vi "encoder_test_3mode_2motor_v1.vi"() -> ()   [LabVIEW 2014]
uses:
  <vilib>/rvi/FXPMathLib/FxpSinAndCos/subVIs/nifxpmath_SinAndCos_SimConfig.ctl
  <vilib>/rvi/Emulation/niFpgaGetClockAttributes.vi
  <vilib>/rvi/Emulation/niFpgaSctlEmulationGetInTimedLoop.vi
  <vilib>/rvi/Emulation/niFpgaEmulationReportErrorSimple.vi
  <vilib>/rvi/eio/common/nirviEmuTemplateMethod_errors.vi
  <vilib>/rvi/Emulation/niFpgaProcessEmulError.vi
  <vilib>/rvi/Emulation/niFpgaCriticalErrorInLSC.vi
  <vilib>/rvi/FXPMathLib/FxpSinAndCos/simVIs/DllFxpSinAndCosTemp_sub.vi
  <vilib>/rvi/interface/RandomDataEmulation/nirviRandomDataMultiElementFPGAFIFO.vi
  <instcachedir>/0/nirviRandomDataMultiElementFPGAFIFO_AD0CFC12EF974623A9C2E4184BC062B2.lvgen/nirviRandomDataMultiElementFPGAFIFO_AD0CFC12EF974623A9C2E4184BC062B2_020.vi
  <vilib>/rvi/interface/RandomDataEmulation/niFpgaRandomDataHandleErrors.vi
  <vilib>/eio/EIONode/EIONode.xnode
  <vilib>/rvi/FXPMathLib/FxpMul/XNode/nifxpmath_Multiplier.xnode
  <vilib>/rvi/FXPMathLib/FxpSinAndCos/XNode/nifxpmath_SinAndCos.xnode
  <vilib>/rvi/Analysis/measure/butterworth/XNode/niFpgaButterworthFilter.xnode
  <vilib>/rvi/FXPMathLib/FxpSub/XNode/nifxpmath_Sub.xnode
  <vilib>/rvi/FXPMathLib/FxpAdd/XNode/nifxpmath_Add.xnode
  <vilib>/rvi/DataTransferAndStorage/Container/XNode/niFpgaContainer.xnode
  <vilib>/rvi/interface/RandomDataEmulation/nirviRandomDataFpgaMultiElementTemplate.vi
  <vilib>/rvi/FXPMathLib/sim/FxpSim.dll
panel:
  out "Dy_d (mm/s)":fxp<+,64,32>
  out "omega_y (rad/s)":fxp<+/-,64,35>
  in  "Velocity Estimation_y":i16(ring) items=["Step", "Ramp", "Sine"]
  out "Dy_d (T)":fxp<+/-,46,10>
  out "mt 2":u32
  out "omega_y (T)":fxp<+/-,20,9>
  out "omega_y (M)":fxp<+/-,64,30>
  out "Dy_d (M)":fxp<+/-,64,27>
  in  "Dy_d_M_Tc (mSec)":u32 format="%#_6f"
  out "omega_y(M_avg)":fxp<+/-,64,35>
  out "Dy_d (M_avg)":fxp<+,64,32>
  in  "Dy_d_M_avg_Tc (uSec)":u32 caption="Count(uSec)"
  out "rad_y(NrTheta)":fxp<+/-,48,33>
  out "Dy (mm)":fxp<+/-,56,32>
  out "Encoder Position_y":i32
  in  "Encoder Reset_y":bool
  out "omega_p (M_avg)":fxp<+/-,64,35>
  out "Dp_d (M_avg)":fxp<+/-,64,32>
  in  "Dp_d_M_avg_Tc (uSec)":u32 caption="D_d_M_avg_Tc (uSec)"
  out "omega_p (M)":fxp<+/-,64,30>
  out "Dp_d (M)":fxp<+/-,64,27>
  in  "Dp_d_M_Tc (mSec)":u32 format="%#_6f"
  out "Dp_d (T)":fxp<+/-,46,10>
  out "omega_p(T)":fxp<+/-,20,9>
  in  "Velocity Estimation_p":i16(ring) items=["M_avg method", "M method", "T method"]
  out "Dpr_ramp":fxp<+/-,64,30>
  out "Dpr_slope":fxp<+/-,33,17>
  in  "Dpr_time":fxp<+/-,16,11>
  out "Dpr_sin":fxp<+/-,28,11>
  out "Dpr_sin_d":fxp<+/-,64,16>
  out "Dpr_sin_dd":fxp<+/-,64,25>
  out "Sin omega_p":fxp<+/-,41,8>
  in  "Sin offset_p":fxp<+/-,27,10>
  in  "Sin magnitude_p":fxp<+/-,11,8>
  in  "Sin wave frequency_p (Hz)":fxp<+/-,21,5>
  out "Time now (s)":fxp<+,52,14>
  out "Dpr":fxp<+/-,64,31>
  in  "Dpr_end":fxp<+/-,16,11>
  in  "Command type_p":i16(ring) items=["Step", "Ramp", "Sine"]
  out "Dp_i":fxp<+/-,34,18>
  in  "Dp_tolorence":fxp<+/-,14,3>
  in  "Ki_p":fxp<+/-,20,6>
  out "Dp_error":fxp<+/-,24,11>
  in  "Direction":bool
  out "Fmr_p":fxp<+/-,64,31>
  in  "Kd_p":fxp<+/-,20,8>
  in  "Kp_p":fxp<+/-,20,12>
  in  "scaled coefficients_Dp_dd":i32[](array[numeric])=[780119100, 146811362]
  out "Dp_dd":fxp<+/-,36,29>
  in  "Ini coe.":bool
  out "va_p":fxp<+/-,38,8>
  out "vb_p":fxp<+/-,38,8>
  in  "stop motor_p":bool
  out "vq_p":fxp<+/-,20,5> format="%.57g"
  out "vd_p":fxp<+/-,20,5>
  out "Dp_d (mm/s)":fxp<+/-,32,12>
  out "mt":u32
  out "omega_p (rad/s)":fxp<+/-,32,18>
  in  "mt0":u32
  out "Dp (mm)":fxp<+/-,22,7>
  out "rad_p(NrTheta)":fxp<+/-,33,18>
  out "Encoder Position_p":i32
  in  "Encoder Reset_p":bool
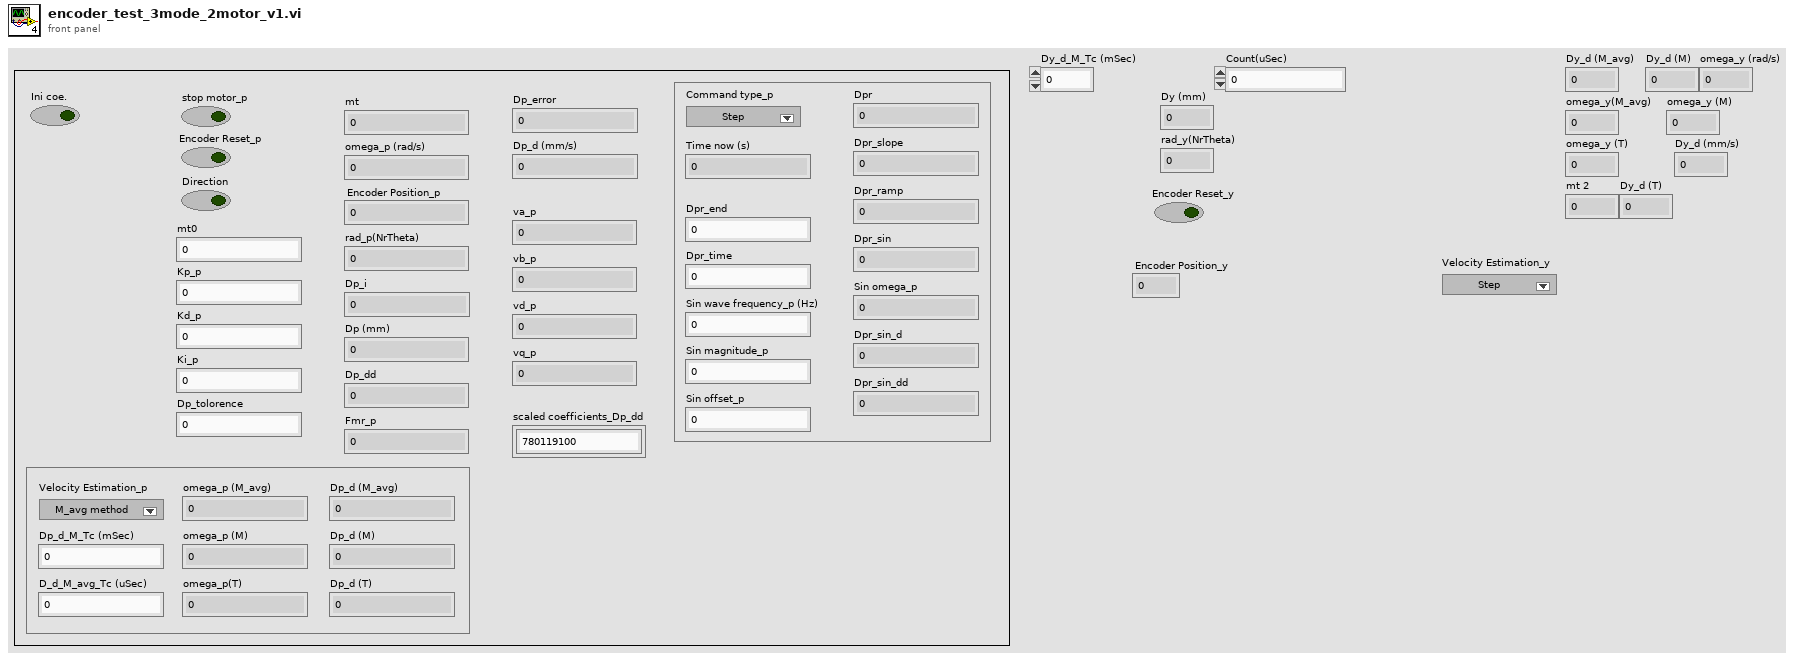
[diagram p1: front panel]
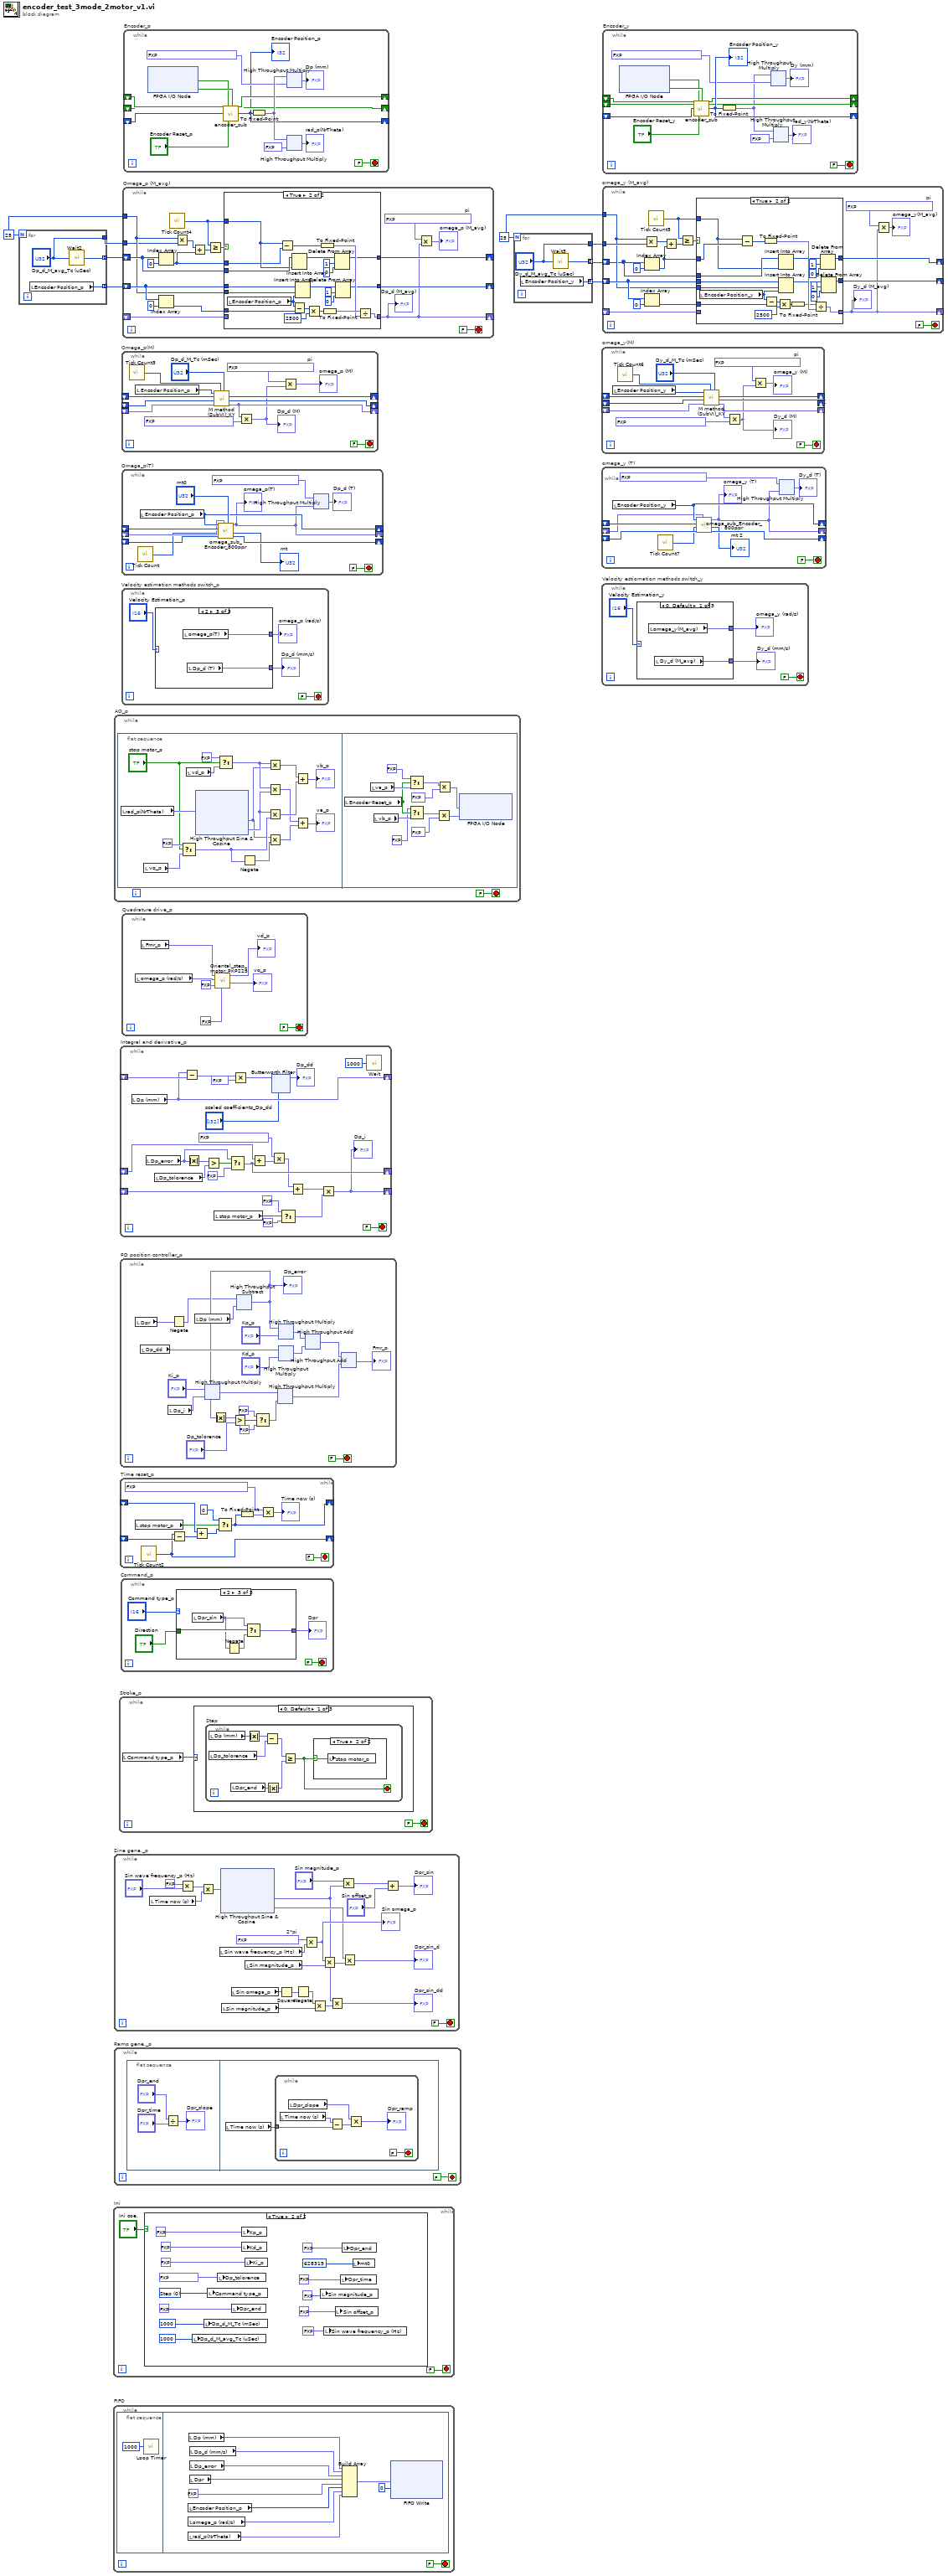
[diagram p0: block diagram]
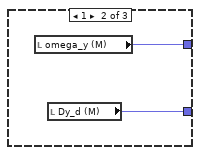
[diagram p2: hidden frame]
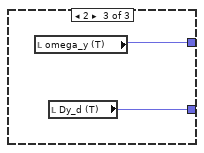
[diagram p3: hidden frame]
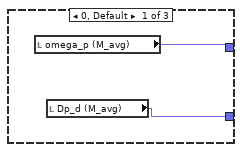
[diagram p6: hidden frame]
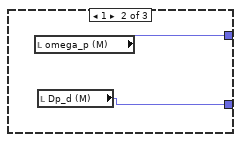
[diagram p7: hidden frame]
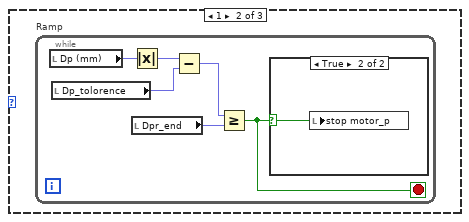
[diagram p9: hidden frame]
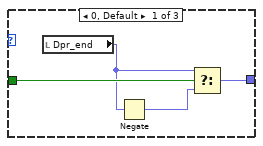
[diagram p12: hidden frame]
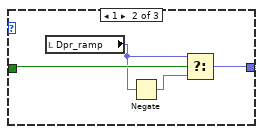
[diagram p13: hidden frame]
diagram:
  w4 = 25
  w8 = 25
  n1 = for {
    N: w8 -> [_]
    tunnel: ["Dp_d_M_avg_Tc (uSec)"] -> w5
    tunnel: [w10] -> w7 mode=indexing
    tunnel: [w9] -> w6 mode=indexing
    n2 = local read "Encoder Position_p"() -> (w9:i32)
    n3 = call "Wait2"("Count(uSec)"="Dp_d_M_avg_Tc (uSec)") -> ("Tick Count(uSec)"=w10:u32)
  }
  n4 = while "Ini" {
    stop <- FALSE stop-if-true
    n5 = case shown="True" "Ini coe." {
      frame False {
      }
      frame True {
        w21 = i16 0 items=["Step", "Ramp", "Sine"] ("Command type")
        n6 = local write "Dp_d_M_avg_Tc (uSec)"(u32 1000 ("D_d_M_avg_Tc (uSec)")) -> ()
        n7 = local write "Dp_d_M_Tc (mSec)"(u32 1000 ("D_d_M_Tc (uSec)")) -> ()
        n8 = local write "Command type_p"(w21) -> ()
        n9 = local write "Dp_tolorence"(fxp<+/-,14,3> 0.009765625 ("D_tolorence")) -> ()
        n10 = local write "Dpr_end"(fxp<+/-,16,11> 20.0 ("Dr_end")) -> ()
        n11 = local write "Kp_p"(fxp<+/-,20,12> 10.0 ("Kp")) -> ()
        n12 = local write "Kd_p"(fxp<+/-,20,8> 2.0 ("Kd")) -> ()
        n13 = local write "Ki_p"(fxp<+/-,20,6> 8.0 ("D_i")) -> ()
        n14 = local write "Sin magnitude_p"(fxp<+/-,11,8> 20.0 ("Sin magnitude")) -> ()
        n15 = local write "Sin wave frequency_p (Hz)"(fxp<+/-,21,5> 0.5 ("Sin wave frequency (Hz)")) -> ()
        n16 = local write "Sin offset_p"(fxp<+/-,27,10> 0.0 ("Sin offset")) -> ()
        n17 = local write "Dpr_time"(fxp<+/-,16,11> 5.0 ("Dr_time")) -> ()
        n18 = local write "Dpr_end"(fxp<+/-,11,7> 20.0 ("Fmr")) -> ()
        n19 = local write "mt0"(u32 628319 ("mt0")) -> ()
      }
    }
  }
  n20 = while "FIFO" {
    stop <- FALSE stop-if-true
    n21 = flat-sequence {
      frame #0 {
        n22 = call "Loop Timer"("Count(uSec)"=u32 1000) -> ()  [unwired: 1 out]
      }
      frame #1 {
        n23 = local read "Encoder Position_p"() -> (w33:i32)
        n24 = local read "omega_p (rad/s)"() -> (w32:fxp<+/-,32,18>)
        n25 = local read "rad_p(NrTheta)"() -> (w31:fxp<+/-,33,18>)
        n26 = local read "Dp (mm)"() -> (w37:fxp<+/-,22,7>)
        n27 = local read "Dp_d (mm/s)"() -> (w36:fxp<+/-,32,12>)
        n28 = local read "Dp_error"() -> (w35:fxp<+/-,24,11>)
        n29 = local read "Dpr"() -> (w34:fxp<+/-,64,31>)
        n30 = Build Array(w37, w36, w35, w34, fxp<+/-,64,32> 0.0 ("element"), w33, w32, w31) -> (w38:fxp<+/-,64,32>[])
        n31 = xnode ("FIFO Write")("Element"=w38, "Timeout"=0) -> ()  [unwired: 1 in, 2 out]
      }
    }
  }
  n32 = while "Sine gene._p" {
    stop <- FALSE stop-if-true
    w57 = fxp<+,20,3> 6.2831878662109375  # 2*pi
    n33 = local read "Time now (s)"() -> (w60:fxp<+,52,14>)
    n34 = Multiply(x=fxp<+,1,2> 2.0, y="Sin wave frequency_p (Hz)") -> (x*y=w61:fxp<+/-,21,6>)
    n35 = Multiply(x=w61, y=w60) -> (x*y=w41:fxp<+/-,64,20>)
    n36 = local read "Sin wave frequency_p (Hz)"() -> (w56:fxp<+/-,21,5>)
    n37 = xnode "High Throughput Sine & Cosine"("x (pi)"=w41) -> ("sin(x)"=w45:fxp<+/-,16,2>, "cos(x)"=w52:fxp<+/-,16,2>)
    n38 = local read "Sin magnitude_p"() -> (w47:fxp<+/-,11,8>)
    n39 = local read "Sin omega_p"() -> (w48:fxp<+/-,41,8>)
    n40 = local read "Sin magnitude_p"() -> (w51:fxp<+/-,11,8>)
    n41 = Square(x=w48) -> (x^2=w49:fxp<+,64,14>)
    n42 = Negate(x=w49) -> (-x=w46:fxp<+/-,64,15>)
    n43 = Multiply(x=w57, y=w56) -> (x*y=w53:fxp<+/-,41,8>)
    "Sin omega_p" <- w53
    n44 = Multiply(x=w46, y=w47) -> (x*y=w50:fxp<+/-,64,23>)
    n45 = Multiply(x=w53, y=w51) -> (x*y=w58:fxp<+/-,51,15>)
    n46 = Multiply(x=w45, y=w50) -> (x*y=→"Dpr_sin_dd":fxp<+/-,64,25>)
    n47 = Multiply(x="Sin magnitude_p", y=w45) -> (x*y=w59:fxp<+/-,27,10>)
    n48 = Multiply(x=w52, y=w58) -> (x*y=→"Dpr_sin_d":fxp<+/-,64,16>)
    n49 = Add(x=w59, y="Sin offset_p") -> (x+y=→"Dpr_sin":fxp<+/-,28,11>)
  }
  n50 = while "Ramp gene._p" {
    stop <- FALSE stop-if-true
    n51 = flat-sequence {
      frame #0 {
        n52 = Divide(x="Dpr_end", y="Dpr_time") -> (x/y=→"Dpr_slope":fxp<+/-,33,17>)
      }
      frame #1 {
        n53 = local read "Time now (s)"() -> (w98:fxp<+,52,14>)
        n54 = while {
          tunnel: w98 -> [w104]
          stop <- FALSE stop-if-true
          n55 = local read "Time now (s)"() -> (w101:fxp<+,52,14>)
          n56 = local read "Dpr_slope"() -> (w102:fxp<+/-,33,17>)
          n57 = Subtract(x=w101, y=w104) -> (x-y=w103:fxp<+/-,53,15>)
          n58 = Multiply(x=w102, y=w103) -> (x*y=→"Dpr_ramp":fxp<+/-,64,30>)
        }
      }
    }
  }
  n59 = while "AO_p" {
    stop <- FALSE stop-if-true
    n60 = flat-sequence {
      frame #0 {
        n61 = local read "rad_p(NrTheta)"() -> (w121:fxp<+/-,33,18>)
        n62 = local read "vq_p"() -> (w119:fxp<+/-,20,5>)
        n63 = Select(t=fxp<+,20,5> 0.0, s="stop motor_p", f=w119) -> (s? t:f=w116:fxp<+/-,21,6>)
        n64 = local read "vd_p"() -> (w120:fxp<+/-,20,5>)
        n65 = xnode "High Throughput Sine & Cosine"("x (pi)"=w121) -> ("sin(x)"=w112:fxp<+/-,17,2>, "cos(x)"=w114:fxp<+/-,17,2>)
        n66 = Select(t=fxp<+,20,5> 0.0, s="stop motor_p", f=w120) -> (s? t:f=w113:fxp<+/-,21,6>)
        n67 = Negate(x=w116) -> (-x=w115:fxp<+/-,21,6>)
        n68 = Multiply(x=w113, y=w112) -> (x*y=w111:fxp<+/-,37,7>)
        n69 = Multiply(x=w113, y=w114) -> (x*y=w109:fxp<+/-,37,7>)
        n70 = Multiply(x=w114, y=w116) -> (x*y=w110:fxp<+/-,37,7>)
        n71 = Multiply(x=w112, y=w115) -> (x*y=w108:fxp<+/-,37,7>)
        n72 = Add(x=w111, y=w110) -> (x+y=→"vb_p":fxp<+/-,38,8>)
        n73 = Add(x=w109, y=w108) -> (x+y=→"va_p":fxp<+/-,38,8>)
      }
      frame #1 {
        n74 = local read "Encoder Reset_p"() -> (w155:bool)
        n75 = local read "va_p"() -> (w157:fxp<+/-,38,8>)
        n76 = local read "vb_p"() -> (w156:fxp<+/-,38,8>)
        n77 = Select(t=fxp<+/-,20,5> 5.0 ("y"), s=w155, f=w157) -> (s? t:f=w158:fxp<+/-,38,8>)
        n78 = Select(t=fxp<+/-,20,5> 0.0 ("y"), s=w155, f=w156) -> (s? t:f=w159:fxp<+/-,38,8>)
        n79 = Multiply(x=w159, y=fxp<+/-,20,5> -0.5) -> (x*y=w163:fxp<+/-,57,12>)
        n80 = Multiply(x=w158, y=fxp<+/-,20,5> -0.5) -> (x*y=w162:fxp<+/-,57,12>)
        n81 = xnode "FPGA I/O Node"("Mod8/AO0"=w162, "Mod8/AO1"=w163) -> ()  [unwired: 2 in, 2 out]
      }
    }
  }
  n82 = while "Stroke_p" {
    stop <- FALSE stop-if-true
    n83 = local read "Command type_p"() -> (w165:i16)
    n84 = case shown="0, Default" w165 {
      frame 0, Default {
        n85 = while "Step" {
          stop <- w166 stop-if-true
          n86 = local read "Dp_tolorence"() -> (w168:fxp<+/-,14,3>)
          n87 = local read "Dp (mm)"() -> (w170:fxp<+/-,22,7>)
          n88 = local read "Dpr_end"() -> (w172:fxp<+/-,16,11>)
          n89 = Absolute Value(x=w170) -> (abs(x)=w169:fxp<+,22,7>)
          n90 = Subtract(x=w169, y=w168) -> (x-y=w167:fxp<+/-,23,8>)
          n91 = Absolute Value(x=w172) -> (abs(x)=w171:fxp<+,16,11>)
          n92 = Greater Or Equal?(x=w167, y=w171) -> (x >= y?=w166:bool)
          n93 = case shown="True" w166 {
            selector: w166 -> [_ w173]
            frame False {
            }
            frame True {
              n94 = local write "stop motor_p"(w173) -> ()
            }
          }
        }
      }
      frame 1 {
        n95 = while "Ramp" {
          stop <- w174 stop-if-true
          n96 = local read "Dp (mm)"() -> (w176:fxp<+/-,22,7>)
          n97 = local read "Dp_tolorence"() -> (w178:fxp<+/-,14,3>)
          n98 = Absolute Value(x=w176) -> (abs(x)=w177:fxp<+,22,7>)
          n99 = local read "Dpr_end"() -> (w175:fxp<+/-,16,11>)
          n100 = Subtract(x=w177, y=w178) -> (x-y=w179:fxp<+/-,23,8>)
          n101 = Greater Or Equal?(x=w179, y=w175) -> (x >= y?=w174:bool)
          n102 = case shown="True" w174 {
            selector: w174 -> [_ w180]
            frame False {
            }
            frame True {
              n103 = local write "stop motor_p"(w180) -> ()
            }
          }
        }
      }
      frame 2 {
      }
    }
  }
  n104 = while "Integral and derivative_p" {
    shift-right: [w201] -> _
    shift-left: _ -> [w205]
    shift-right: [w191] -> _
    shift-left: _ -> [w192]
    shift-right: [w181] -> _
    shift-left: _ -> [w185]
    stop <- FALSE stop-if-true
    n105 = local read "Dp (mm)"() -> (w201:fxp<+/-,22,7>)
    n106 = local read "Dp_error"() -> (w193:fxp<+/-,24,11>)
    n107 = local read "Dp_tolorence"() -> (w196:fxp<+/-,14,3>)
    n108 = Subtract(x=w201, y=w205) -> (x-y=w204:fxp<+/-,23,8>)
    n109 = Absolute Value(x=w193) -> (abs(x)=w197:fxp<+,24,11>)
    n110 = Greater?(x=w197, y=w196) -> (0:w195:bool)
    n111 = local read "stop motor_p"() -> (w188:bool)
    n112 = Select(t=w193, s=w195, f=fxp<+,24,11> 0.0) -> (s? t:f=w191:fxp<+/-,25,12>)
    n113 = Multiply(x=w204, y=fxp<+/-,33,13> 1000.0) -> (x*y=w202:fxp<+/-,55,20>)
    n114 = Add(x=w192, y=w191) -> (x+y=w190:fxp<+/-,26,13>)
    n115 = Multiply(x=fxp<+/-,30,12> 0.000499725341796875, y=w190) -> (x*y=w184:fxp<+/-,55,24>)
    n116 = xnode "Butterworth Filter"("input data"=w202, "scaled coefficients"="scaled coefficients_Dp_dd") -> ("output data"=→"Dp_dd":fxp<+/-,36,24>)  [unwired: 1 in]
    n117 = Select(t=fxp<+,1,1> 0.0, s=w188, f=fxp<+,1,1> 1.0) -> (s? t:f=w182:fxp<+,1,1>)
    n118 = Add(x=w184, y=w185) -> (x+y=w183:fxp<+/-,32,16>)
    n119 = Multiply(x=w183, y=w182) -> (x*y=w181:fxp<+/-,32,16>)
    "Dp_i" <- w181
    n120 = call "Wait"("Count(uSec)"=u32 1000) -> ()  [unwired: 1 out]
  }
  n121 = while "PD position controller_p" {
    stop <- FALSE stop-if-true
    n122 = local read "Dpr"() -> (w216:fxp<+/-,64,31>)
    n123 = local read "Dp_dd"() -> (w232:fxp<+/-,36,29>)
    n124 = local read "Dp_i"() -> (w227:fxp<+/-,34,18>)
    n125 = Negate(x=w216) -> (-x=w215:fxp<+/-,64,32>)
    n126 = local read "Dp (mm)"() -> (w236:fxp<+/-,22,7>)
    n127 = xnode ("High Throughput Multiply")("x"="Ki_p", "y"=w227) -> ("x*y"=w221:fxp<+/-,54,24>)
    n128 = xnode "High Throughput Subtract"("x"=w215, "y"=w236) -> ("x-y"=w225:fxp<+/-,64,33>)
    "Dp_error" <- w225
    n129 = Absolute Value(x=w225) -> (abs(x)=w226:fxp<+,64,33>)
    n130 = Greater?(x=w226, y="Dp_tolorence") -> (0:w224:bool)
    n131 = Select(t=fxp<+,10,2> 1.0, s=w224, f=fxp<+,10,2> 0.0) -> (s? t:f=w220:fxp<+,10,2>)
    n132 = xnode ("High Throughput Multiply")("x"=w221, "y"=w220) -> ("x*y"=w217:fxp<+/-,64,26>)
    n133 = xnode ("High Throughput Multiply")("x"=w225, "y"="Kp_p") -> ("x*y"=w234:fxp<+/-,64,45>)
    n134 = xnode ("High Throughput Multiply")("x"=w232, "y"="Kd_p") -> ("x*y"=w233:fxp<+/-,56,37>)
    n135 = xnode ("High Throughput Add")("x"=w234, "y"=w233) -> ("x+y"=w218:fxp<+/-,64,46>)
    n136 = xnode ("High Throughput Add")("x"=w218, "y"=w217) -> ("x+y"=→"Fmr_p":fxp<+/-,64,47>)
  }
  n137 = while "Time reset_p" {
    shift-right: [w240] -> _
    shift-left: _ -> [w247]
    shift-right: [w242] -> _
    shift-left: _ -> [w243]
    stop <- FALSE stop-if-true
    n138 = local read "stop motor_p"() -> (w245:bool)
    n139 = call "Tick Count2"() -> ("Tick Count(uSec)"=w242:u32)
    n140 = Subtract(x=w242, y=w243) -> (x-y=w248:u32)
    n141 = Add(x=w247, y=w248) -> (x+y=w246:u32)
    n142 = Select(t=u32 0, s=w245, f=w246) -> (s? t:f=w240:u32)
    n143 = To Fixed-Point(number=w240) -> (fixed-point=w239:fxp<+,32,32>)  [unwired: 1 in]
    n144 = Multiply(x=fxp<+,20,-18> 1.0000003385357559e-06, y=w239) -> (x*y=→"Time now (s)":fxp<+,52,14>)
  }
  n145 = while "Command_p" {
    stop <- FALSE stop-if-true
    n146 = case shown="2" "Command type_p" {
      tunnel: [w253 w257 w261] -> w251
      tunnel: "Direction" -> [w256 w260 w264]
      frame 0, Default {
        n147 = local read "Dpr_end"() -> (w255:fxp<+/-,16,11>)
        n148 = Negate(x=w255) -> (-x=w254:fxp<+/-,17,12>)
        n149 = Select(t=w255, s=w256, f=w254) -> (s? t:f=w253:fxp<+/-,17,12>)
      }
      frame 1 {
        n150 = local read "Dpr_ramp"() -> (w258:fxp<+/-,64,30>)
        n151 = Negate(x=w258) -> (-x=w259:fxp<+/-,64,31>)
        n152 = Select(t=w258, s=w260, f=w259) -> (s? t:f=w257:fxp<+/-,64,31>)
      }
      frame 2 {
        n153 = local read "Dpr_sin"() -> (w262:fxp<+/-,28,11>)
        n154 = Negate(x=w262) -> (-x=w263:fxp<+/-,27,10>)
        n155 = Select(t=w262, s=w264, f=w263) -> (s? t:f=w261:fxp<+/-,28,11>)
      }
    }
    "Dpr" <- w251
  }
  n156 = while "Omega_p(M)" {
    shift-right: [w276] -> _
    shift-left: _ -> [w277]
    shift-right: [w272] -> _
    shift-left: _ -> [w273]
    shift-right: [w270] -> _
    shift-left: _ -> [w271]
    stop <- FALSE stop-if-true
    w267 = fxp<+/-,27,3> 3.1415926218032837  # pi
    n157 = call "Tick Count3"() -> ("Tick Count(mSec)"=w275:u32)
    n158 = local read "Encoder Position_p"() -> (w278:i32)
    n159 = call "M method (SubVI)_KY.vi"("Tc (mSec)"="Dp_d_M_Tc (mSec)", "Tick Count (mSec)"=w275, "Encoder velocity_pre (pulse/s)"=w271, "Shift Register in 2"=w273, "Shift Register in 1"=w277, "Encoder pulses"=w278) -> ("Encoder velocity (pulse/s)"=w270:fxp<+/-,64,32>, "Shift Register out 2"=w272:i32, "Shift Register out 1"=w276:u32)  [unwired: 3 in]
    n160 = Multiply(x=w270, y=fxp<+/-,20,-5> 0.002499997615814209) -> (x*y=w268:fxp<+/-,64,27>)
    "Dp_d (M)" <- w268
    n161 = Multiply(x=w267, y=w268) -> (x*y=→"omega_p (M)":fxp<+/-,64,30>)
  }
  n162 = while "Omega_p(T)" {
    shift-right: [w288] -> _
    shift-left: _ -> [w289]
    shift-right: [w281] -> _
    shift-left: _ -> [w287]
    shift-right: [w284] -> _
    shift-left: _ -> [w285]
    stop <- FALSE stop-if-true
    n163 = call "Tick Count"() -> ("Tick Count(Ticks)"=w286:u32)
    n164 = local read "Encoder Position_p"() -> (w288:i32)
    n165 = call "omega_sub_Encoder_800ppr.vi"("mt0"="mt0", "omega_pre"=w287, "ticks_m_pre"=w285, "ticks"=w286, "count_pre"=w289, "count"=w288) -> ("ticks_m"=w284:u32, "mt"=→"mt":u32, "omega"=w281:fxp<+/-,20,9>)  [unwired: 3 in]
    "omega_p(T)" <- w281
    n166 = xnode ("High Throughput Multiply")("x"=fxp<+/-,26,1> 0.3183099031448364, "y"=w281) -> ("x*y"=→"Dp_d (T)":fxp<+/-,46,10>)
  }
  n167 = while "Velocity estimation methods switch_p" {
    stop <- FALSE stop-if-true
    n168 = case shown="2" "Velocity Estimation_p" {
      tunnel: [w296 w298 w300] -> w293
      tunnel: [w295 w297 w299] -> w292
      frame 0, Default {
        n169 = local read "omega_p (M_avg)"() -> (w296:fxp<+/-,64,35>)
        n170 = local read "Dp_d (M_avg)"() -> (w295:fxp<+/-,64,32>)
      }
      frame 1 {
        n171 = local read "omega_p (M)"() -> (w298:fxp<+/-,64,30>)
        n172 = local read "Dp_d (M)"() -> (w297:fxp<+/-,64,27>)
      }
      frame 2 {
        n173 = local read "omega_p(T)"() -> (w300:fxp<+/-,20,9>)
        n174 = local read "Dp_d (T)"() -> (w299:fxp<+/-,46,10>)
      }
    }
    "Dp_d (mm/s)" <- w292
    "omega_p (rad/s)" <- w293
  }
  n175 = while "Quadrature drive_p" {
    stop <- FALSE stop-if-true
    n176 = local read "omega_p (rad/s)"() -> (w303:fxp<+/-,32,18>)
    n177 = local read "Fmr_p"() -> (w301:fxp<+/-,64,31>)
    n178 = call "Oriental_step_motor_PKP225.vi"("F_Threshold"=fxp<+,12,12> 10.0, "dFmr"=fxp<+/-,25,15> 0.0, "omega"=w303, "Fmr"=w301) -> ("vq_F"=→"vq_p":fxp<+/-,20,5>, "vd_F"=→"vd_p":fxp<+/-,20,5>)  [unwired: 6 in]
  }
  n179 = while "Omega_p (M_avg)" {
    tunnel: w8 -> [w319]
    shift-right: [w312] -> _
    shift-left: w7 -> [w323]
    shift-right: [w311] -> _
    shift-left: _ -> [w314]
    shift-right: [w313] -> _
    shift-left: w6 -> [w322]
    tunnel: w5 -> [w316]
    stop <- FALSE stop-if-true
    w310 = fxp<+/-,27,3> 3.1415926218032837  # pi
    n180 = Index Array(array=w323, index=0) -> (element=w317:u32)
    n181 = Index Array(array=w322, index=0) -> (element=w318:i32)
    n182 = call "Tick Count4"() -> ("Tick Count(uSec)"=w320:u32)
    n183 = Multiply(x=w319, y=w316) -> (x*y=w324:u32)
    n184 = Add(x=w324, y=w317) -> (x+y=w321:u32)
    n185 = Greater Or Equal?(x=w320, y=w321) -> (x >= y?=w315:bool)
    n186 = case shown="True" w315 {
      tunnel: w323 -> [w329 w346]
      tunnel: w322 -> [w328 w345]
      tunnel: w320 -> [_ w338]
      tunnel: w319 -> [_ w344]
      tunnel: w318 -> [_ w342]
      tunnel: w317 -> [_ w337]
      tunnel: w314 -> [w327 _]
      tunnel: [w328 w332] -> w313
      tunnel: [w329 w331] -> w312
      tunnel: [w327 w330] -> w311
      frame False {
      }
      frame True {
        n187 = local read "Encoder Position_p"() -> (w343:i32)
        n188 = Subtract(x=w338, y=w337) -> (x-y=w335:u32)
        n189 = Insert Into Array(array=w346, new element=w338) -> (w347:u32[])  [unwired: 1 in]
        n190 = Subtract(x=w343, y=w342) -> (x-y=w341:i32)
        n191 = Insert Into Array(array=w345, index=w344, new element=w343) -> (w348:i32[])
        n192 = Multiply(x=w341, y=2500) -> (x*y=w339:i32)
        n193 = To Fixed-Point(number=w335) -> (fixed-point=w333:fxp<+,32,32>)  [unwired: 1 in]
        n194 = To Fixed-Point(number=w339) -> (fixed-point=w334:fxp<+/-,32,32>)  [unwired: 1 in]
        n195 = Delete From Array(array=w347, length=1, index=0) -> (array with subset deleted=w331:u32[])  [unwired: 1 out]
        n196 = Delete From Array(array=w348, length=1, index=0) -> (array with subset deleted=w332:i32[])  [unwired: 1 out]
        n197 = Divide(x=w334, y=w333) -> (x/y=w330:fxp<+/-,64,32>)
      }
    }
    "Dp_d (M_avg)" <- w311
    n198 = Multiply(x=w310, y=w311) -> (x*y=→"omega_p (M_avg)":fxp<+/-,64,35>)
  }
  n199 = while "Encoder_p" {
    shift-right: [w358] -> _
    shift-left: _ -> [w360]
    shift-right: [w357] -> _
    shift-left: _ -> [w359]
    shift-right: [w355] -> _
    shift-left: _ -> [w356]
    stop <- FALSE stop-if-true
    n200 = xnode "FPGA I/O Node"() -> ("Mod4/DI3"=w365:bool, "Mod4/DI4"=w366:bool)  [unwired: 2 in, 2 out]
    n201 = call "encoder_sub.vi"("A_pre"=w360, "B_pre"=w359, "Encoder Position_pre"=w356, "A input"=w365, "Encoder Position Reset"="Encoder Reset_p", "B input"=w366) -> ("A"=w358:bool, "B"=w357:bool, "Encoder Position (Counts)"=w355:i32)  [unwired: 19 in]
    "Encoder Position_p" <- w355
    n202 = To Fixed-Point(number=w355) -> (fixed-point=w363:fxp<+/-,32,32>)  [unwired: 1 in]
    n203 = xnode ("High Throughput Multiply")("x"=w363, "y"=fxp<+/-,24,0> 0.002499997615814209) -> ("x*y"=→"Dp (mm)":fxp<+/-,56,32>)
    n204 = xnode ("High Throughput Multiply")("x"=w363, "y"=fxp<+/-,24,0> 0.125) -> ("x*y"=→"rad_p(NrTheta)":fxp<+/-,56,32>)
  }
  n205 = for {
    N: w4 -> [_]
    tunnel: ["Dy_d_M_avg_Tc (uSec)"] -> w3
    tunnel: [w368] -> w1 mode=indexing
    tunnel: [w367] -> w2 mode=indexing
    n206 = local read "Encoder Position_y"() -> (w367:i32)
    n207 = call "Wait3"("Count(uSec)"="Dy_d_M_avg_Tc (uSec)") -> ("Tick Count(uSec)"=w368:u32)
  }
  n208 = while "omega_y(M)" {
    shift-right: [w376] -> _
    shift-left: _ -> [w380]
    shift-right: [w377] -> _
    shift-left: _ -> [w379]
    shift-right: [w375] -> _
    shift-left: _ -> [w378]
    stop <- FALSE stop-if-true
    w372 = fxp<+/-,27,3> 3.1415926218032837  # pi
    n209 = local read "Encoder Position_y"() -> (w383:i32)
    n210 = call "Tick Count6"() -> ("Tick Count(mSec)"=w382:u32)
    n211 = call "M method (SubVI)_KY.vi"("Tc (mSec)"="Dy_d_M_Tc (mSec)", "Tick Count (mSec)"=w382, "Encoder velocity_pre (pulse/s)"=w378, "Shift Register in 2"=w379, "Shift Register in 1"=w380, "Encoder pulses"=w383) -> ("Encoder velocity (pulse/s)"=w375:fxp<+/-,64,32>, "Shift Register out 2"=w377:i32, "Shift Register out 1"=w376:u32)  [unwired: 3 in]
    n212 = Multiply(x=w375, y=fxp<+/-,20,-5> 0.002499997615814209) -> (x*y=w373:fxp<+/-,64,27>)
    "Dy_d (M)" <- w373
    n213 = Multiply(x=w372, y=w373) -> (x*y=→"omega_y (M)":fxp<+/-,64,30>)
  }
  n214 = while "omega_y (T)" {
    shift-right: [w393] -> _
    shift-left: _ -> [w392]
    shift-right: [w387] -> _
    shift-left: _ -> [w391]
    shift-right: [w394] -> _
    shift-left: _ -> [w390]
    stop <- FALSE stop-if-true
    n215 = local read "Encoder Position_y"() -> (w393:i32)
    n216 = call "Tick Count7"() -> ("Tick Count(Ticks)"=w389:u32)
    n217 = call "omega_sub_Encoder_800ppr.vi"("omega_pre"=w391, "ticks_m_pre"=w390, "ticks"=w389, "count_pre"=w392, "count"=w393) -> ("ticks_m"=w394:u32, "mt"=→"mt 2":u32, "omega"=w387:fxp<+/-,20,9>)  [unwired: 4 in]
    "omega_y (T)" <- w387
    n218 = xnode "High Throughput Multiply"("x"=fxp<+/-,26,1> 0.3183099031448364, "y"=w387) -> ("x*y"=→"Dy_d (T)":fxp<+/-,46,10>)
  }
  n219 = while "Velocity estiomation methods switch_y" {
    stop <- FALSE stop-if-true
    n220 = case shown="0, Default" "Velocity Estimation_y" {
      tunnel: [w400 w401 w404] -> w397
      tunnel: [w399 w402 w403] -> w396
      frame 0, Default {
        n221 = local read "omega_y(M_avg)"() -> (w400:fxp<+/-,64,35>)
        n222 = local read "Dy_d (M_avg)"() -> (w399:fxp<+,64,32>)
      }
      frame 1 {
        n223 = local read "omega_y (M)"() -> (w401:fxp<+/-,64,30>)
        n224 = local read "Dy_d (M)"() -> (w402:fxp<+/-,64,27>)
      }
      frame 2 {
        n225 = local read "omega_y (T)"() -> (w404:fxp<+/-,20,9>)
        n226 = local read "Dy_d (T)"() -> (w403:fxp<+/-,46,10>)
      }
    }
    "omega_y (rad/s)" <- w397
    "Dy_d (mm/s)" <- w396
  }
  n227 = while "omega_y (M_avg)" {
    tunnel: w4 -> [w414]
    tunnel: w3 -> [w420]
    shift-right: [w410] -> _
    shift-left: w1 -> [w411]
    shift-right: [w409] -> _
    shift-left: w2 -> [w415]
    shift-right: [w407] -> _
    shift-left: _ -> [w412]
    stop <- FALSE stop-if-true
    w408 = fxp<+/-,27,3> 3.1415926218032837  # pi
    n228 = Multiply(x=w414, y=w420) -> (x*y=w419:u32)
    n229 = Index Array(array=w411, index=0) -> (element=w416:u32)
    n230 = Index Array(array=w415, index=0) -> (element=w413:i32)
    n231 = call "Tick Count5"() -> ("Tick Count(uSec)"=w417:u32)
    n232 = Add(x=w419, y=w416) -> (x+y=w423:u32)
    n233 = Greater Or Equal?(x=w417, y=w423) -> (x >= y?=w418:bool)
    n234 = case shown="True" w418 {
      tunnel: w417 -> [_ w446]
      tunnel: w416 -> [_ w447]
      tunnel: w415 -> [w425 w436]
      tunnel: w414 -> [_ w437]
      tunnel: w413 -> [_ w438]
      tunnel: w412 -> [w424 _]
      tunnel: w411 -> [w426 w448]
      tunnel: [w426 w429] -> w410
      tunnel: [w425 w428] -> w409
      tunnel: [w424 w427] -> w407
      frame False {
      }
      frame True {
        n235 = local read "Encoder Position_y"() -> (w439:i32)
        n236 = Subtract(x=w446, y=w447) -> (x-y=w445:u32)
        n237 = To Fixed-Point(number=w445) -> (fixed-point=w444:fxp<+,32,32>)  [unwired: 1 in]
        n238 = Subtract(x=w439, y=w438) -> (x-y=w440:i32)
        n239 = Multiply(x=w440, y=u32 2500) -> (x*y=w442:u32)
        n240 = Insert Into Array(array=w448, new element=w446) -> (w434:u32[])  [unwired: 1 in]
        n241 = Insert Into Array(array=w436, index=w437, new element=w439) -> (w435:i32[])
        n242 = To Fixed-Point(number=w442) -> (fixed-point=w443:fxp<+,32,32>)  [unwired: 1 in]
        n243 = Divide(x=w443, y=w444) -> (x/y=w427:fxp<+,64,32>)
        n244 = Delete From Array(array=w434, length=1, index=0) -> (array with subset deleted=w429:u32[])  [unwired: 1 out]
        n245 = Delete From Array(array=w435, length=1, index=0) -> (array with subset deleted=w428:i32[])  [unwired: 1 out]
      }
    }
    "Dy_d (M_avg)" <- w407
    n246 = Multiply(x=w408, y=w407) -> (x*y=→"omega_y(M_avg)":fxp<+/-,64,35>)
  }
  n247 = while "Encoder_y" {
    shift-right: [w457] -> _
    shift-left: _ -> [w455]
    shift-right: [w458] -> _
    shift-left: _ -> [w456]
    shift-right: [w461] -> _
    shift-left: _ -> [w460]
    stop <- FALSE stop-if-true
    n248 = xnode "FPGA I/O Node"() -> ("Mod4/DI0"=w462:bool, "Mod4/DI1"=w463:bool)  [unwired: 2 in, 2 out]
    n249 = call "encoder_sub.vi"("A_pre"=w455, "B_pre"=w456, "Encoder Position_pre"=w460, "A input"=w462, "Encoder Position Reset"="Encoder Reset_y", "B input"=w463) -> ("A"=w457:bool, "B"=w458:bool, "Encoder Position (Counts)"=w461:i32)  [unwired: 19 in]
    "Encoder Position_y" <- w461
    n250 = To Fixed-Point(number=w461) -> (fixed-point=w452:fxp<+/-,32,32>)  [unwired: 1 in]
    n251 = xnode "High Throughput Multiply"("x"=w452, "y"=fxp<+/-,24,0> 0.002499997615814209) -> ("x*y"=→"Dy (mm)":fxp<+/-,56,32>)
    n252 = xnode "High Throughput Multiply"("x"=w452, "y"=fxp<+/-,16,1> 0.125) -> ("x*y"=→"rad_y(NrTheta)":fxp<+/-,48,33>)
  }
